vi "checkDAQAnalogValue.vi"(1 "Reference":dbl[](array[numeric])=[1.0, 1.0], 2 "Array":dbl[](array[numeric])=[5.6581196784973145, 6.761904716491699]) -> (0 "thresholded analog inputs":bool[](array[boolean])=[TRUE, TRUE])   [LabVIEW 2011]
uses:
  GlobalDAQ.vi
panel:
  in  "DetectedActiveTime (ms)":u32=500
  out "millisecond timer value":u32=618982556
  in  "index high":i32=1
  in  "index low":i32
  in  "LB0ActiveTime (ms)":u32=1000
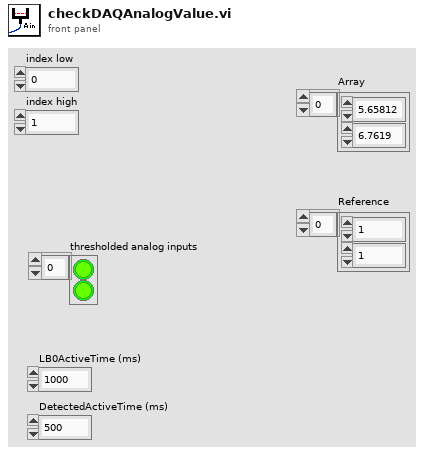
[diagram p1: front panel]
types:
  T1 = cluster{"det 0":bool, "det time 0":u32, "det 1":bool, "det time 1":u32, "detected":bool, "detection time":u32}
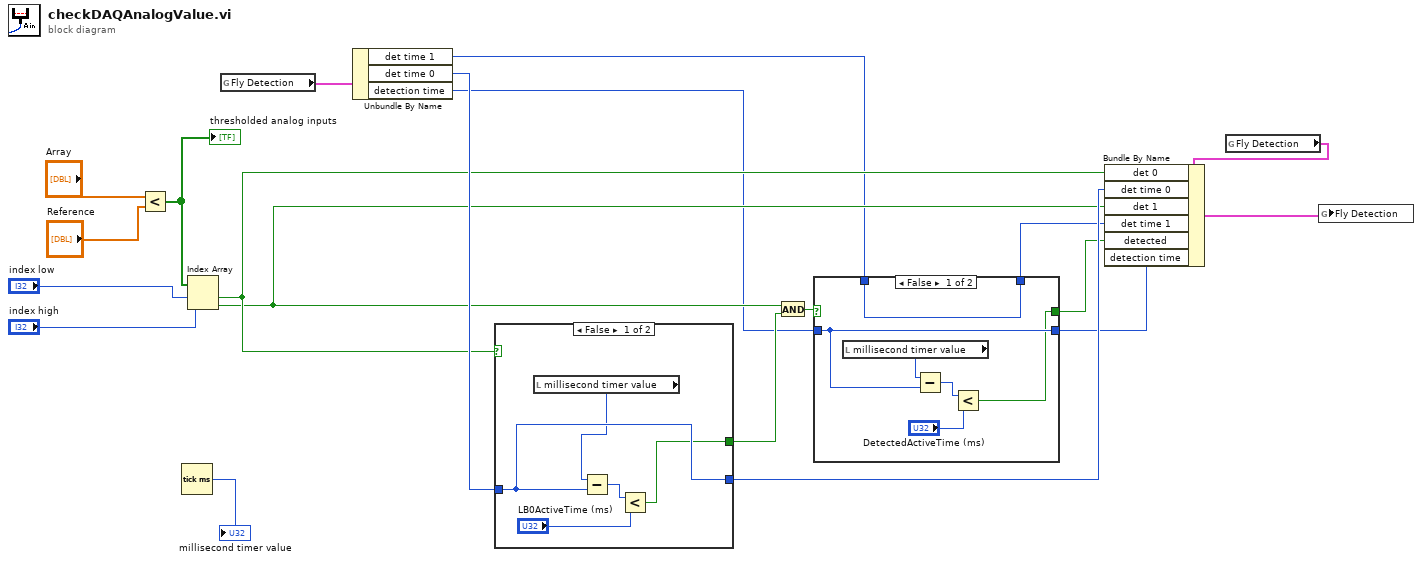
[diagram p0: block diagram]
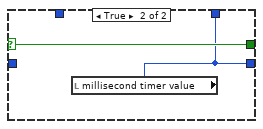
[diagram p2: hidden frame]
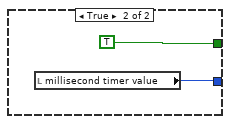
[diagram p3: hidden frame]
diagram:
  n1 = Less?(x="Array", y="Reference") -> (x < y?=w19:bool[])
  "thresholded analog inputs" <- w19
  n2 = Tick Count (ms)() -> (millisecond timer value=→"millisecond timer value":u32)
  n3 = Index Array(array=w19, index #1="index low", index #2="index high") -> (element #1=w11:bool, element #2=w10:bool)
  n4 = global read "GlobalDAQ.vi" "Fly Detection"() -> (w14:T1)
  n5 = Unbundle By Name(w14) -> ("det time 1"=w2:u32, "det time 0"=w13:u32, "detection time"=w8:u32)
  n6 = case shown="False" w11 {
    tunnel: [w22 TRUE] -> w18
    tunnel: [w23 w26] -> w12
    tunnel: w13 -> [w23 _]
    frame False {
      n7 = local read "millisecond timer value"() -> (w21:u32)
      n8 = Subtract(x=w21, y=w23) -> (x-y=w25:u32)
      n9 = Less?(x=w25, y="LB0ActiveTime (ms)") -> (x < y?=w22:bool)
    }
    frame True {
      n10 = local read "millisecond timer value"() -> (w26:u32)
    }
  }
  n11 = And(x=w10, y=w18) -> (x .and. y?=w7:bool)
  n12 = case shown="False" w7 {
    selector: w7 -> [_ w35]
    tunnel: [w31 w34] -> w9
    tunnel: w8 -> [w31 _]
    tunnel: [w29 w35] -> w6
    tunnel: [w28 w34] -> w3
    tunnel: w2 -> [w28 _]
    frame False {
      n13 = local read "millisecond timer value"() -> (w32:u32)
      n14 = Subtract(x=w32, y=w31) -> (x-y=w33:u32)
      n15 = Less?(x=w33, y="DetectedActiveTime (ms)") -> (x < y?=w29:bool)
    }
    frame True {
      n16 = local read "millisecond timer value"() -> (w34:u32)
    }
  }
  n17 = global read "GlobalDAQ.vi" "Fly Detection"() -> (w15:T1)
  n18 = Bundle By Name(cluster=w15, "det 0"=w11, "det time 0"=w12, "det 1"=w10, "det time 1"=w3, "detected"=w6, "detection time"=w9) -> (w4:T1)
  n19 = global write "GlobalDAQ.vi" "Fly Detection"(w4) -> ()
